vi "Distance Between Colors.vi"(8 "error in (no error)":errorcluster, 10 "Color 2":u32(colorbox), 11 "Color 1":u32(colorbox)) -> (0 "error out":errorcluster, 3 "Distance":dbl)   [LabVIEW 2015, in "ColorSelector.lvclass"]
doc: "This VI uses the RGB values of two colors to represent points in a 3-D space and then determines the distance between the points.\n<b> </b> <b> </b>\n©2017 Q Software Innovations, LLC (QSI)\nwritten by Quentin Alldredge\nproduced in LabVIEW 2015\n\nsupport@qsoftwareinnovations.com\nwww.qsoftwareinnovations.com\n\nAll rights reserved.\n\nRedistribution and use in source and binary forms, with or without modification, are permitted provided that the following conditions are met:\n\n * Redistributions of source code must retain the above copyright notice, this list of conditions and the following disclaimer.\n * Redistributions in binary form must reproduce the above copyright notice, this list of conditions and the following disclaimer in the documentation and/or other materials provided with the distribution.\n * Neither the name of Q Software Innovations, LLC. nor the names of its contributors may be used to endorse or promote products derived from this software without specific prior written permission.\n\nTHIS SOFTWARE IS PROVIDED BY THE COPYRIGHT HOLDERS AND CONTRIBUTORS \"AS IS\" AND ANY EXPRESS OR IMPLIED WARRANTIES, INCLUDING, BUT NOT LIMITED TO, THE IMPLIED WARRANTIES OF MERCHANTABILITY AND FITNESS FOR A PARTICULAR PURPOSE ARE DISCLAIMED. IN NO EVENT SHALL THE COPYRIGHT OWNER OR CONTRIBUTORS BE LIABLE FOR ANY DIRECT, INDIRECT, INCIDENTAL, SPECIAL, EXEMPLARY, OR CONSEQUENTIAL DAMAGES (INCLUDING, BUT NOT LIMITED TO, PROCUREMENT OF SUBSTITUTE GOODS OR SERVICES; LOSS OF USE, DATA, OR PROFITS; OR BUSINESS INTERRUPTION) HOWEVER CAUSED AND ON ANY THEORY OF LIABILITY, WHETHER IN CONTRACT, STRICT LIABILITY, OR TORT (INCLUDING NEGLIGENCE OR OTHERWISE) ARISING IN ANY WAY OUT OF THE USE OF THIS SOFTWARE, EVEN IF ADVISED OF THE POSSIBILITY OF SUCH DAMAGE."
uses:
  ColorSelector.lvclass
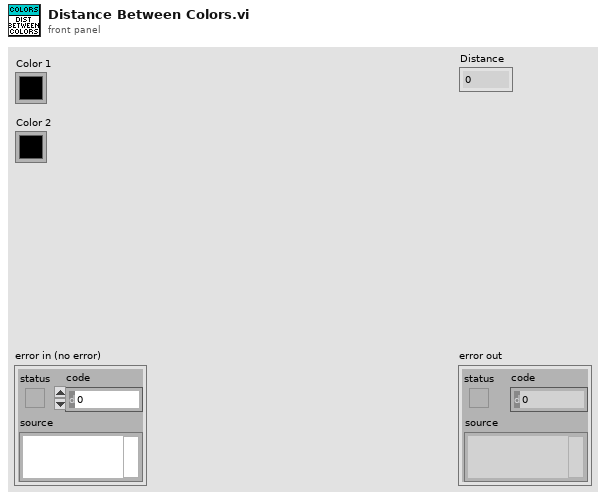
[diagram p1: front panel]
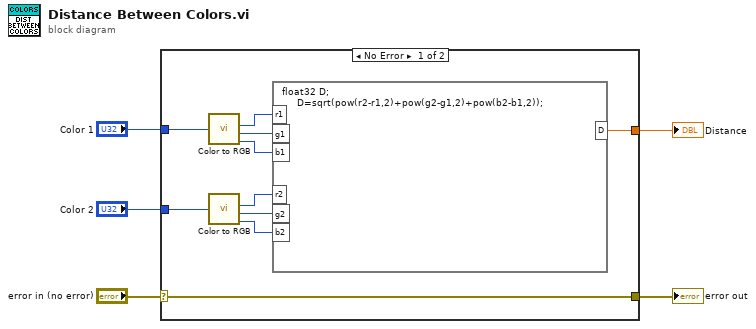
[diagram p0: block diagram]
diagram:
  n1 = case shown="No Error" "error in (no error)" {
    selector: "error in (no error)" -> [w15 w16]
    tunnel: [w15 w16] -> w4
    tunnel: "Color 1" -> [w14 _]
    tunnel: [w10 _] -> w2
    tunnel: "Color 2" -> [w9 _]
    frame No Error {
      n2 = call <vilib>:"Color to RGB.vi"("Color"=w14) -> ("R"=w13:u8, "G"=w12:u8, "B"=w11:u8)  [unwired: 1 out]
      n3 = call <vilib>:"Color to RGB.vi"("Color"=w9) -> ("R"=w7:u8, "G"=w8:u8, "B"=w6:u8)  [unwired: 1 out]
      n4 = formula code="float32 D;\n     D=sqrt(pow(r2-r1,2)+pow(g2-g1,2)+pow(b2-b1,2));"("r1"=w13, "g1"=w12, "b1"=w11, "r2"=w7, "g2"=w8, "b2"=w6) -> ("D"=w10:sgl)
    }
    frame Error {
    }
  }
  "error out" <- w4
  "Distance" <- w2
